vi "Close.vi"(8 "error in (no error)":errorcluster, 11 "DataTable in":refnum<class "DataTable.lvclass">) -> (0 "error out":errorcluster, 3 "DataTable out":refnum<class "DataTable.lvclass">)   [LabVIEW 2013, in "DataGrid.lvlib" / "DataTable.lvclass"]
uses:
  DataTable.lvclass
  DataTable.lvclass/DataTable.ctl
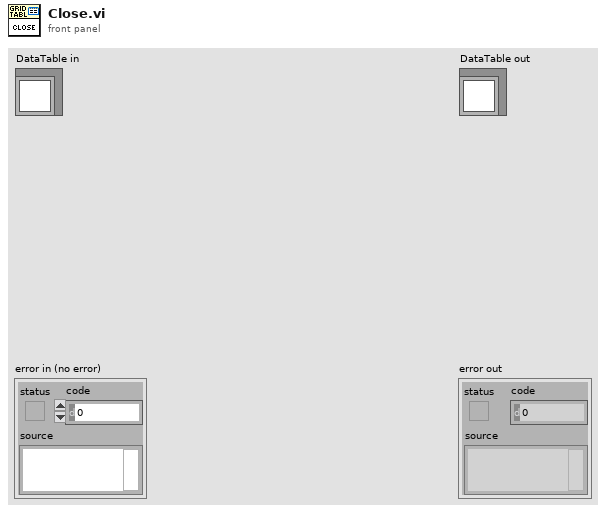
[diagram p1: front panel]
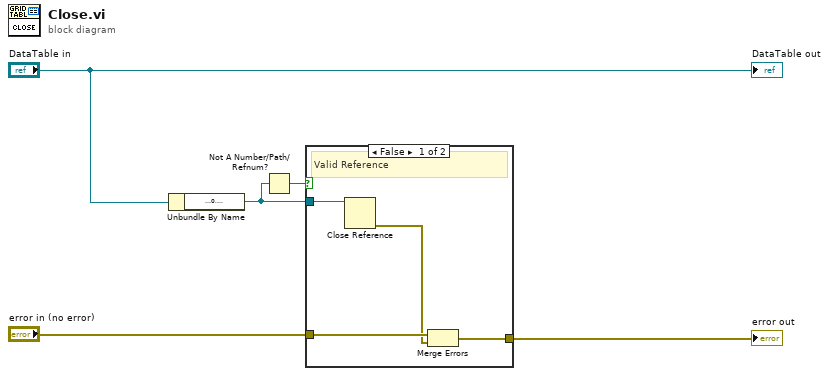
[diagram p0: block diagram]
diagram:
  n1 = Unbundle By Name("DataTable in") -> ("DataTable"=w2:refnum<k24>)
  n2 = Not A Number/Path/Refnum?(number/path/refnum=w2) -> (NaN/Path/Refnum?=w1:bool)
  n3 = case shown="False" w1 {
    tunnel: "error in (no error)" -> [w9 w10]
    tunnel: [w8 w10] -> w3
    tunnel: w2 -> [w6 _]
    frame False {
      # "Valid Reference"
      n4 = Close Reference(reference=w6) -> (error out=w7:errorcluster)  [unwired: 1 in]
      n5 = Merge Errors(w9, w7) -> (w8:errorcluster)
    }
    frame True {
      # "Probably never initialised. Ignore."
      # "Not A Valid Reference"
    }
  }
  "error out" <- w3
  "DataTable out" <- "DataTable in"
